vi "Host_HoppingScan(ZFPGAWithin).vi"() -> ()   [LabVIEW 2014]
uses:
  <vilib>/Native 3D Graph/xcontrol/3DPC_SurfacePlot.xctl
  <vilib>/Instr/_visa.llb/VISA Configure Serial Port (Instr).vi
  <vilib>/FPGAPlugInAG/PCIe-7851R/niLvFpga_Open_PCIe-7851R.vi
  <vilib>/rvi/interface/common/dynamic/niFpgaDynamicAddResources.vi
  <vilib>/Utility/error.llb/Error Cluster From Error Code.vi
  <vilib>/rvi/errors/niLvFpgaAdjustHostInterfaceError.vi
  <vilib>/FPGAPlugInAG/Dynamic/niLvFpga_Close_Dynamic.vi
  <vilib>/rvi/interface/nirviOpenFPGA/nirviOpenFPGA.xnode
  FPGA Bitfiles/XZFPGAWithinHopp_FPGATarget_FGPAHoppingStep(_pqW261ZDZNw.lvbitx
  <vilib>/rvi/interface/nirviReadWriteControl/nirviReadWriteControl.xnode
  <vilib>/rvi/interface/nirviMethod/nirviMethod.xnode
  <vilib>/rvi/interface/nirviCloseFPGA/nirviCloseFPGA.xnode
  <vilib>/rvi/interface/Simulation/niFpgaSimulationCallBeginRW.vi
  <vilib>/FPGAPlugInAG/Dynamic/niLvFpga_ReadFifo_Dynamic.vi
  <vilib>/rvi/errors/niLvFpgaMergeErrorWithErrorCode.vi
  NiFpgaLv.dll
panel:
  out "YPresPos":dbl
  out "YPresNum":i32
  in  "Relative?":bool
  in  "RelativeWithdraw":i16
  in  "YStepLen um":dbl
  in  "YInitPos um":dbl
  in  "YNum":i16
  in  "BottomSleep us":i16
  in  "UpperSleep us":i16
  out "3D Graph":refnum<class "Base Datatype.lvclass">[](xcontrol)
  out "ZRealTimePos":i16(graph)
  out "XPresPos":dbl
  in  "Stop":bool
  out "XPresNum":i32
  in  "ZOffset":i16
  out "ERR?":string
  in  "XNum":i16
  in  "XInitPos um":dbl
  in  "XStepLen um":dbl
  in  "RoughX":refnum<visa-resource-name>
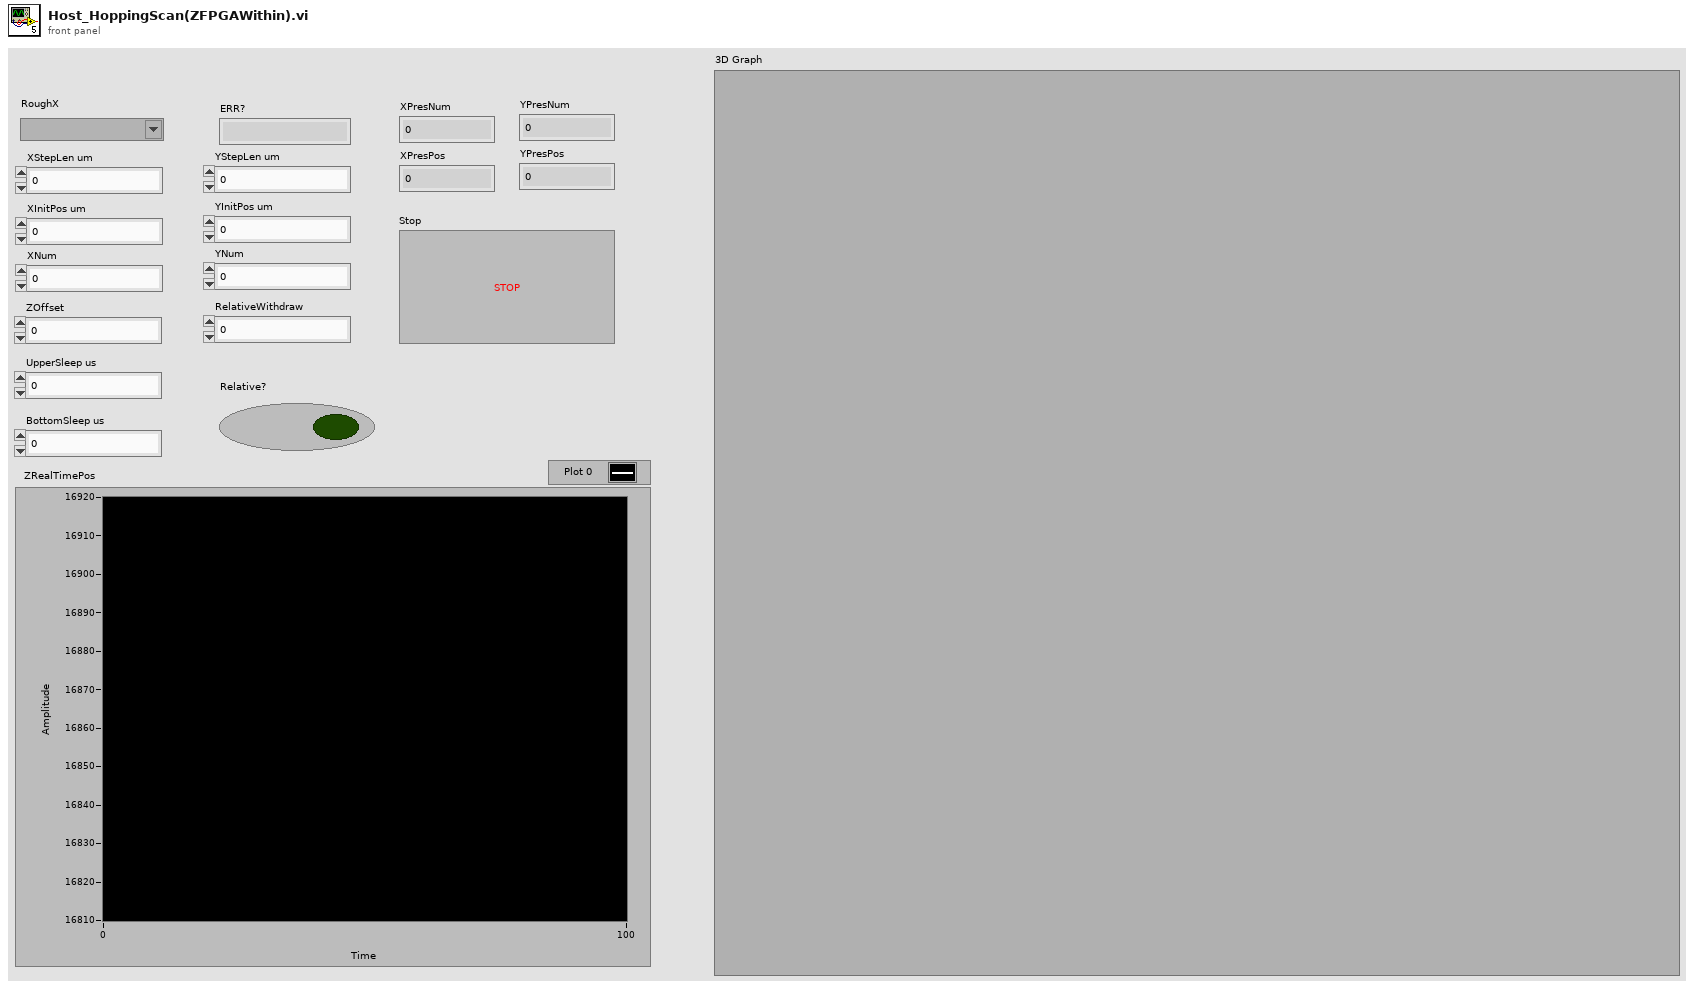
[diagram p1: front panel]
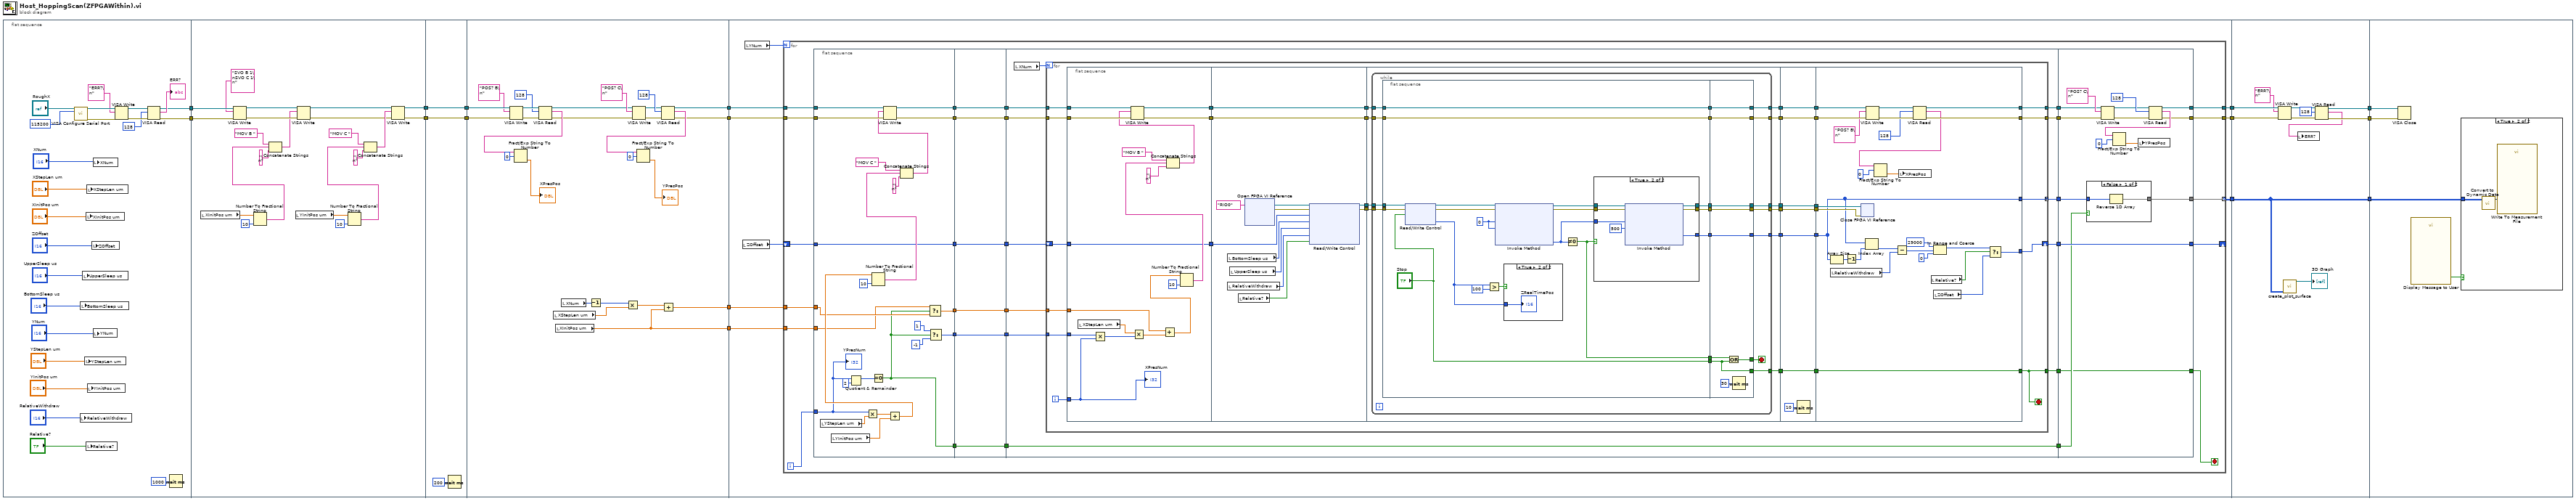
[diagram p0: block diagram]
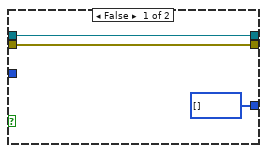
[diagram p3: hidden frame]
diagram:
  n1 = flat-sequence {
    tunnel: [w27] -> w16
    tunnel: [w26] -> w15
    tunnel: w16 -> [w60]
    tunnel: w15 -> [w59]
    tunnel: [w41] -> w12
    tunnel: [w40] -> w11
    tunnel: w12 -> [w63]
    tunnel: [w63] -> w10
    tunnel: w11 -> [w62]
    tunnel: [w62] -> w8
    tunnel: w10 -> [w89]
    tunnel: [w72] -> w9
    tunnel: w8 -> [w88]
    tunnel: [w71] -> w7
    tunnel: [w66] -> w2
    tunnel: [w65] -> w1
    tunnel: w9 -> [w98]
    tunnel: w7 -> [w97]
    tunnel: [w96] -> w14
    tunnel: [w95] -> w13
    tunnel: [w94] -> w6
    tunnel: w2 -> [w92]
    tunnel: w1 -> [w91]
    tunnel: w14 -> [w357]
    tunnel: w13 -> [w356]
    tunnel: w6 -> [w347]
    tunnel: [w351] -> w5
    tunnel: [w350] -> w4
    tunnel: [w347] -> w3
    tunnel: w5 -> [w361]
    tunnel: w4 -> [w360]
    tunnel: w3 -> [w358]
    frame #0 {
      n2 = call-poly "VISA Configure Serial Port"("VISA resource name"="RoughX", "baud rate (9600)"=u32 115200) -> ("VISA resource name out"=w37:refnum<visa-resource-name>, "error out"=w36:errorcluster)  [unwired: 12 in]
      n3 = local write "RelativeWithdraw"("RelativeWithdraw") -> ()
      n4 = local write "BottomSleep us"("BottomSleep us") -> ()
      n5 = local write "UpperSleep us"("UpperSleep us") -> ()
      n6 = local write "YStepLen um"("YStepLen um") -> ()
      n7 = local write "XInitPos um"("XInitPos um") -> ()
      n8 = local write "Relative?"("Relative?") -> ()
      n9 = local write "XStepLen um"("XStepLen um") -> ()
      n10 = local write "YInitPos um"("YInitPos um") -> ()
      n11 = local write "ZOffset"("ZOffset") -> ()
      n12 = local write "XNum"("XNum") -> ()
      n13 = local write "YNum"("YNum") -> ()
      n14 = VISA Write(VISA resource name=w37, write buffer="ERR?\n", error in (no error)=w36) -> (VISA resource name out=w35:refnum<visa-resource-name>, error out=w34:errorcluster)  [unwired: 1 out]
      n15 = VISA Read(VISA resource name=w35, byte count=u32 128, error in (no error)=w34) -> (VISA resource name out=w27:refnum<visa-resource-name>, read buffer=→"ERR?":string, error out=w26:errorcluster)  [unwired: 1 out]
      n16 = Wait (ms)(milliseconds to wait=u32 1000) -> ()  [unwired: 1 out]
    }
    frame #1 {
      n17 = local read "XInitPos um"() -> (w53:dbl)
      n18 = VISA Write(VISA resource name=w60, write buffer="SVO B 1\nSVO C 1\n", error in (no error)=w59) -> (VISA resource name out=w57:refnum<visa-resource-name>, error out=w56:errorcluster)  [unwired: 1 out]
      n19 = Number To Fractional String(number=w53, precision (6)=i16 10) -> (F-format string=w51:string)  [unwired: 2 in]
      n20 = Concatenate Strings("MOV B " ("string"), w51, "\n" ("string")) -> (w54:string)
      n21 = local read "YInitPos um"() -> (w46:dbl)
      n22 = VISA Write(VISA resource name=w57, write buffer=w54, error in (no error)=w56) -> (VISA resource name out=w43:refnum<visa-resource-name>, error out=w42:errorcluster)  [unwired: 1 out]
      n23 = Number To Fractional String(number=w46, precision (6)=i16 10) -> (F-format string=w48:string)  [unwired: 2 in]
      n24 = Concatenate Strings("MOV C " ("string"), w48, "\n" ("string")) -> (w44:string)
      n25 = VISA Write(VISA resource name=w43, write buffer=w44, error in (no error)=w42) -> (VISA resource name out=w41:refnum<visa-resource-name>, error out=w40:errorcluster)  [unwired: 1 out]
    }
    frame #2 {
      n26 = Wait (ms)(milliseconds to wait=u32 200) -> ()  [unwired: 1 out]
    }
    frame #3 {
      n27 = VISA Write(VISA resource name=w89, write buffer="POS? B\n", error in (no error)=w88) -> (VISA resource name out=w87:refnum<visa-resource-name>, error out=w86:errorcluster)  [unwired: 1 out]
      n28 = VISA Read(VISA resource name=w87, byte count=u32 128, error in (no error)=w86) -> (VISA resource name out=w74:refnum<visa-resource-name>, read buffer=w83:string, error out=w73:errorcluster)  [unwired: 1 out]
      n29 = Fract/Exp String To Number(string=w83, offset=0) -> (number=→"XPresPos":dbl)  [unwired: 2 in, 1 out]
      n30 = local read "XStepLen um"() -> (w68:dbl)
      n31 = local read "XInitPos um"() -> (w65:dbl)
      n32 = local read "XNum"() -> (w70:i16)
      n33 = Decrement(x=w70) -> (x-1=w69:i16)
      n34 = Multiply(x=w69, y=w68) -> (x*y=w67:dbl)
      n35 = VISA Write(VISA resource name=w74, write buffer="POS? C\n", error in (no error)=w73) -> (VISA resource name out=w75:refnum<visa-resource-name>, error out=w76:errorcluster)  [unwired: 1 out]
      n36 = VISA Read(VISA resource name=w75, byte count=u32 128, error in (no error)=w76) -> (VISA resource name out=w72:refnum<visa-resource-name>, read buffer=w79:string, error out=w71:errorcluster)  [unwired: 1 out]
      n37 = Fract/Exp String To Number(string=w79, offset=0) -> (number=→"YPresPos":dbl)  [unwired: 2 in, 1 out]
      n38 = Add(x=w67, y=w65) -> (x+y=w66:dbl)
    }
    frame #4 {
      n39 = local read "ZOffset"() -> (w90:i16)
      n40 = local read "YNum"() -> (w93:i16)
      n41 = for {
        N: w93 -> [_]
        tunnel: [w116] -> w94 mode=indexing
        tunnel: w98 -> [w120]
        tunnel: [w118] -> w96
        tunnel: w97 -> [w119]
        tunnel: [w117] -> w95
        tunnel: w92 -> [w114]
        tunnel: w91 -> [w113]
        shift-right: [w104] -> _
        shift-left: w90 -> [w106]
        i -> [w115]
        stop <- w99 stop-if-true
        n42 = flat-sequence {
          tunnel: w119 -> [w150]
          tunnel: w120 -> [w151]
          tunnel: [w149] -> w127
          tunnel: [w148] -> w126
          tunnel: w115 -> [w138]
          tunnel: w114 -> [w135]
          tunnel: w113 -> [w134]
          tunnel: [w131] -> w111
          tunnel: [w130] -> w109
          tunnel: [w129] -> w108
          tunnel: w106 -> [w129]
          tunnel: [w128] -> w102
          tunnel: [w157] -> w125
          tunnel: [w156] -> w124
          tunnel: w126 -> [w156]
          tunnel: w127 -> [w157]
          tunnel: [w155] -> w112
          tunnel: w111 -> [w155]
          tunnel: [w154] -> w110
          tunnel: w109 -> [w154]
          tunnel: w108 -> [w153]
          tunnel: [w153] -> w107
          tunnel: [w152] -> w103
          tunnel: w102 -> [w152]
          tunnel: [w166] -> w123
          tunnel: [w165] -> w122
          tunnel: [w164] -> w121
          tunnel: w125 -> [w168]
          tunnel: w124 -> [w167]
          tunnel: w112 -> [w163]
          tunnel: w110 -> [w162]
          tunnel: w107 -> [w161]
          tunnel: [w160] -> w105
          tunnel: w103 -> [w159]
          tunnel: [w159] -> w101
          tunnel: [w158] -> w100
          tunnel: [w340] -> w116
          tunnel: [w329] -> w117
          tunnel: [w330] -> w118
          tunnel: w123 -> [w332]
          tunnel: w122 -> [w331]
          tunnel: w121 -> [w341]
          tunnel: w105 -> [w343]
          tunnel: [w343] -> w104
          tunnel: w101 -> [w342]
          tunnel: [w339] -> w99
          tunnel: w100 -> [w339]
          frame #0 {
            n43 = local read "YStepLen um"() -> (w142:dbl)
            n44 = local read "YInitPos um"() -> (w140:dbl)
            n45 = Quotient & Remainder(x=w138, y=2) -> (x-y*floor(x/y)=w136:i32)  [unwired: 1 out]
            n46 = Multiply(x=w138, y=w142) -> (x*y=w141:dbl)
            n47 = Equal To 0?(x=w136) -> (x = 0?=w128:bool)
            n48 = Add(x=w141, y=w140) -> (x+y=w139:dbl)
            n49 = Number To Fractional String(number=w139, precision (6)=i16 10) -> (F-format string=w145:string)  [unwired: 2 in]
            n50 = Concatenate Strings("MOV C " ("string"), w145, "\n" ("string")) -> (w143:string)
            n51 = VISA Write(VISA resource name=w151, write buffer=w143, error in (no error)=w150) -> (VISA resource name out=w149:refnum<visa-resource-name>, error out=w148:errorcluster)  [unwired: 1 out]
            n52 = Select(t=w134, s=w128, f=w135) -> (s? t:f=w131:dbl)
            n53 = Select(t=1 ("y"), s=w128, f=-1 ("y")) -> (s? t:f=w130:i32)
            "YPresNum" <- w138
          }
          frame #1 {
          }
          frame #2 {
            n54 = local read "XNum"() -> (w169:i16)
            n55 = for {
              N: w169 -> [_]
              tunnel: w168 -> [w199]
              tunnel: w167 -> [w198]
              tunnel: [w178] -> w166
              tunnel: [w177] -> w165
              tunnel: [w176] -> w164 mode=concatenating
              tunnel: w163 -> [w175]
              tunnel: w162 -> [w174]
              shift-right: [w171] -> w160
              shift-left: w161 -> [w173]
              tunnel: [w170] -> w158
              i -> [w197]
              stop <- w170 stop-if-true
              n56 = flat-sequence {
                tunnel: w199 -> [w216]
                tunnel: w198 -> [w215]
                tunnel: w197 -> [w206]
                tunnel: [w214] -> w194
                tunnel: [w213] -> w193
                tunnel: w175 -> [w202]
                tunnel: w174 -> [w207]
                tunnel: w173 -> [w200]
                tunnel: [w200] -> w172
                tunnel: [w225] -> w196
                tunnel: [w224] -> w195
                tunnel: w194 -> [w223]
                tunnel: w193 -> [w222]
                tunnel: [w223] -> w192
                tunnel: [w222] -> w191
                tunnel: w172 -> [w219]
                tunnel: w196 -> [w238]
                tunnel: w195 -> [w237]
                tunnel: w192 -> [w236]
                tunnel: w191 -> [w235]
                tunnel: [w234] -> w190
                tunnel: [w233] -> w189
                tunnel: [w232] -> w188
                tunnel: [w231] -> w187
                tunnel: [w230] -> w181
                tunnel: [w229] -> w179
                tunnel: w190 -> [w298]
                tunnel: w189 -> [w297]
                tunnel: w188 -> [w300]
                tunnel: w187 -> [w299]
                tunnel: [w300] -> w186
                tunnel: [w299] -> w185
                tunnel: [w298] -> w184
                tunnel: [w297] -> w183
                tunnel: [w296] -> w182
                tunnel: w181 -> [w296]
                tunnel: [w295] -> w180
                tunnel: w179 -> [w295]
                tunnel: w186 -> [w326]
                tunnel: w185 -> [w325]
                tunnel: w184 -> [w324]
                tunnel: w183 -> [w323]
                tunnel: w182 -> [w312]
                tunnel: w180 -> [w327]
                tunnel: [w327] -> w170
                tunnel: [w318] -> w178
                tunnel: [w317] -> w177
                tunnel: [w312] -> w176
                tunnel: [w302] -> w171
                frame #0 {
                  n57 = local read "XStepLen um"() -> (w204:dbl)
                  n58 = Multiply(x=w207, y=w206) -> (x*y=w205:i32)
                  n59 = Multiply(x=w204, y=w205) -> (x*y=w203:dbl)
                  n60 = Add(x=w202, y=w203) -> (x+y=w201:dbl)
                  n61 = Number To Fractional String(number=w201, precision (6)=i16 10) -> (F-format string=w211:string)  [unwired: 2 in]
                  n62 = Concatenate Strings("MOV B " ("string"), w211, "\n" ("string")) -> (w208:string)
                  n63 = VISA Write(VISA resource name=w216, write buffer=w208, error in (no error)=w215) -> (VISA resource name out=w214:refnum<visa-resource-name>, error out=w213:errorcluster)  [unwired: 1 out]
                  "XPresNum" <- w206
                }
                frame #1 {
                  n64 = local read "BottomSleep us"() -> (w221:i16)
                  n65 = local read "RelativeWithdraw"() -> (w218:i16)
                  n66 = local read "UpperSleep us"() -> (w220:i16)
                  n67 = local read "Relative?"() -> (w217:bool)
                  n68 = xnode "Open FPGA VI Reference"("resource name"=tag "RIO0") -> ("FPGA VI Reference Out"=w227:refnum<k20>, "error out"=w226:errorcluster)  [unwired: 1 in]
                  n69 = xnode "Read/Write Control"("FPGA VI Reference In"=w227, "error in"=w226, "ZOffset"=w219, "BottomSleep us"=w221, "UpperSleep us"=w220, "RelativeWithdraw"=w218, "Relative?"=w217) -> ("FPGA VI Reference Out"=w225:refnum<k20>, "error out"=w224:errorcluster)
                }
                frame #2 {
                  n70 = while {
                    tunnel: w238 -> [w256]
                    tunnel: w237 -> [w255]
                    tunnel: w236 -> [w254]
                    tunnel: w235 -> [w253]
                    tunnel: [w249] -> w230
                    tunnel: [w247] -> w234
                    tunnel: [w245] -> w233
                    tunnel: [w241] -> w232
                    tunnel: [w240] -> w231
                    tunnel: [w239] -> w229
                    stop <- w244 stop-if-true
                    n71 = flat-sequence {
                      tunnel: w256 -> [w274]
                      tunnel: w255 -> [w273]
                      tunnel: w254 -> [w264]
                      tunnel: w253 -> [w263]
                      tunnel: [w267] -> w252
                      tunnel: [w266] -> w251
                      tunnel: [w265] -> w250
                      tunnel: [w264] -> w248
                      tunnel: [w263] -> w246
                      tunnel: [w261] -> w243
                      tunnel: ["Stop"] -> w242
                      tunnel: w252 -> [w288]
                      tunnel: w251 -> [w287]
                      tunnel: w250 -> [w293]
                      tunnel: [w293] -> w249
                      tunnel: w248 -> [w292]
                      tunnel: [w292] -> w247
                      tunnel: w246 -> [w291]
                      tunnel: [w291] -> w245
                      tunnel: [w290] -> w244
                      tunnel: w243 -> [w289]
                      tunnel: w242 -> [w286]
                      tunnel: [w288] -> w241
                      tunnel: [w287] -> w240
                      tunnel: [w286] -> w239
                      frame #0 {
                        w270 = u32 0 ("Number of Elements")
                        n72 = xnode "Read/Write Control"("FPGA VI Reference In"=w274, "error in"=w273, "stop"="Stop") -> ("FPGA VI Reference Out"=w272:refnum<k20>, "error out"=w271:errorcluster, "ZRealPos"=w259:i16)
                        n73 = Greater?(x=w259, y=i16 100) -> (0:w257:bool)
                        n74 = xnode "Invoke Method"("FPGA VI Reference In"=w272, "error in"=w271, "Number of Elements"=w270, "Timeout (ms)"=w270) -> ("FPGA VI Reference Out"=w269:refnum<k20>, "error out"=w268:errorcluster, "Elements Remaining"=w260:u32)  [unwired: 1 out]
                        n75 = case shown="True" w257 {
                          tunnel: w259 -> [_ w275]
                          frame False {
                          }
                          frame True {
                            "ZRealTimePos" <- w275
                          }
                        }
                        n76 = Not Equal To 0?(x=w260) -> (x != 0?=w261:bool)
                        n77 = case shown="True" w261 {
                          tunnel: w269 -> [w278 w285]
                          tunnel: w268 -> [w277 w284]
                          tunnel: [w278 w282] -> w267
                          tunnel: [w277 w281] -> w266
                          tunnel: [i16[] [] ("Data") w280] -> w265
                          tunnel: w260 -> [_ w279]
                          frame False {
                          }
                          frame True {
                            n78 = xnode "Invoke Method"("FPGA VI Reference In"=w285, "error in"=w284, "Number of Elements"=w279, "Timeout (ms)"=500) -> ("FPGA VI Reference Out"=w282:refnum<k20>, "error out"=w281:errorcluster, "Data"=w280:i16[])  [unwired: 1 out]
                          }
                        }
                      }
                      frame #1 {
                        n79 = Or(x=w289, y=w286) -> (x .or. y?=w290:bool)
                        n80 = Wait (ms)(milliseconds to wait=u32 30) -> ()  [unwired: 1 out]
                      }
                    }
                  }
                }
                frame #3 {
                  n81 = Wait (ms)(milliseconds to wait=u32 10) -> ()  [unwired: 1 out]
                }
                frame #4 {
                  n82 = Array Size(array=w312) -> (size(s)=w313:i32)
                  n83 = local read "RelativeWithdraw"() -> (w309:i16)
                  n84 = Decrement(x=w313) -> (x-1=w311:i32)
                  n85 = xnode "Close FPGA VI Reference"("FPGA VI Reference In"=w326, "error in"=w325) -> ()  [unwired: 1 out]
                  n86 = Index Array(array=w312, index=w311) -> (element=w310:i16)
                  n87 = VISA Write(VISA resource name=w324, write buffer="POS? B\n", error in (no error)=w323) -> (VISA resource name out=w321:refnum<visa-resource-name>, error out=w320:errorcluster)  [unwired: 1 out]
                  n88 = Subtract(x=w310, y=w309) -> (x-y=w308:i16)
                  n89 = VISA Read(VISA resource name=w321, byte count=u32 128, error in (no error)=w320) -> (VISA resource name out=w318:refnum<visa-resource-name>, read buffer=w316:string, error out=w317:errorcluster)  [unwired: 1 out]
                  n90 = Fract/Exp String To Number(string=w316, offset=0) -> (number=w314:dbl)  [unwired: 2 in, 1 out]
                  n91 = local write "XPresPos"(w314) -> ()
                  n92 = local read "Relative?"() -> (w303:bool)
                  n93 = In Range and Coerce(upper limit=i16 29000, x=w308, lower limit=i16 0 ("upper limit")) -> (coerced(x)=w305:i16)  [unwired: 1 out]
                  n94 = local read "ZOffset"() -> (w304:i16)
                  n95 = Select(t=w305, s=w303, f=w304) -> (s? t:f=w302:i16)
                }
              }
            }
          }
          frame #3 {
            n96 = case shown="False" w342 {
              tunnel: w341 -> [w345 w346]
              tunnel: [w344 w346] -> w340
              frame False {
                n97 = Reverse 1D Array(array=w345) -> (reversed array=w344:i16[])
              }
              frame True {
              }
            }
            n98 = VISA Write(VISA resource name=w332, write buffer="POS? C\n", error in (no error)=w331) -> (VISA resource name out=w334:refnum<visa-resource-name>, error out=w335:errorcluster)  [unwired: 1 out]
            n99 = VISA Read(VISA resource name=w334, byte count=u32 128, error in (no error)=w335) -> (VISA resource name out=w330:refnum<visa-resource-name>, read buffer=w337:string, error out=w329:errorcluster)  [unwired: 1 out]
            n100 = Fract/Exp String To Number(string=w337, offset=0) -> (number=w328:dbl)  [unwired: 2 in, 1 out]
            n101 = local write "YPresPos"(w328) -> ()
          }
        }
      }
    }
    frame #5 {
      n102 = VISA Write(VISA resource name=w357, write buffer="ERR?\n", error in (no error)=w356) -> (VISA resource name out=w354:refnum<visa-resource-name>, error out=w353:errorcluster)  [unwired: 1 out]
      n103 = call <vilib>:"create_plot_surface.vi"("z matrix"=w347) -> ("plots out"=→"3D Graph":refnum<class "Base Datatype.lvclass">[])  [unwired: 4 in, 6 out]
      n104 = VISA Read(VISA resource name=w354, byte count=u32 128, error in (no error)=w353) -> (VISA resource name out=w351:refnum<visa-resource-name>, read buffer=w349:string, error out=w350:errorcluster)  [unwired: 1 out]
      n105 = local write "ERR?"(w349) -> ()
    }
    frame #6 {
      n106 = VISA Close(VISA resource name=w361, error in (no error)=w360) -> ()  [unwired: 1 out]
      n107 = call "Display Message to User"() -> ("OK"=w359:bool)  [unwired: 10 in, 1 out]
      n108 = case shown="True" w359 {
        tunnel: w358 -> [_ w363]
        frame False {
        }
        frame True {
          n109 = call "Convert to Dynamic Data"("2D Array"=w363) -> ("Dynamic Data Type"=w362:dynamicdata)  [unwired: 3 in]
          n110 = call "Write To Measurement File"("Signals"=w362) -> ()  [unwired: 16 in, 3 out]
        }
      }
    }
  }
